vi "MicronsToPixels.vi"(9 "Scan Settings (um)":T1={"XStart"=-100, "XEnd"=100, "XNum"=250, "YStart"=-100, "YEnd"=100, "YNum"=250, "ZStart"=-50, "ZEnd"=50, "ZNum"=30}, 11 "Microns (X,Y,Z)":dbl[](array[numeric])) -> (3 "Pixels (X,Y,Z)":i32[](array[numeric]))   [LabVIEW 2014]
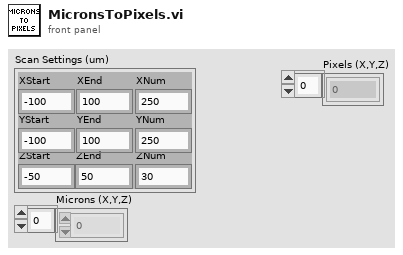
[diagram p1: front panel]
types:
  T1 = cluster{"XStart":i32, "XEnd":i32, "XNum":i32, "YStart":i32, "YEnd":i32, "YNum":i32, "ZStart":i32, "ZEnd":i32, "ZNum":i32}
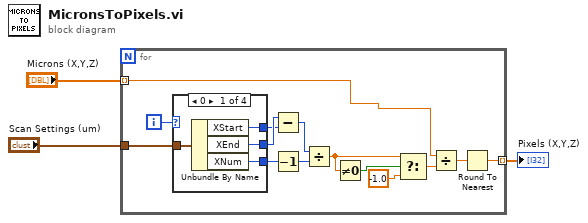
[diagram p0: block diagram]
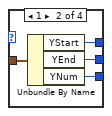
[diagram p2: hidden frame]
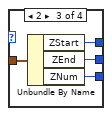
[diagram p3: hidden frame]
diagram:
  n1 = for {
    tunnel: "Scan Settings (um)" -> [w16]
    tunnel: "Microns (X,Y,Z)" -> [w4] mode=indexing
    tunnel: [w10] -> w1 mode=indexing
    i -> [w17]
    n2 = case shown="0" w17 {
      tunnel: w16 -> [w19 w23 w29 _]
      tunnel: [w20 w24 w28 _] -> w15
      tunnel: [w21 w25 w27 _] -> w5
      tunnel: [w18 w22 w26 _] -> w13
      frame 0 {
        n3 = Unbundle By Name(w19) -> ("XStart"=w21:i32, "XEnd"=w20:i32, "XNum"=w18:i32)
      }
      frame 1 {
        n4 = Unbundle By Name(w23) -> ("YStart"=w25:i32, "YEnd"=w24:i32, "YNum"=w22:i32)
      }
      frame 2 {
        n5 = Unbundle By Name(w29) -> ("ZStart"=w27:i32, "ZEnd"=w28:i32, "ZNum"=w26:i32)
      }
      frame Default {
      }
    }
    n6 = Subtract(x=w15, y=w5) -> (x-y=w14:i32)
    n7 = Decrement(x=w13) -> (x-1=w12:i32)
    n8 = Divide(x=w14, y=w12) -> (x/y=w8:dbl)
    n9 = Not Equal To 0?(x=w8) -> (x != 0?=w9:bool)
    n10 = Select(t=w8, s=w9, f=-1.0) -> (s? t:f=w7:dbl)
    n11 = Divide(x=w4, y=w7) -> (x/y=w11:dbl)
    n12 = Round To Nearest(number=w11) -> (nearest integer value=w10:dbl)
  }
  "Pixels (X,Y,Z)" <- w1
